vi "ex_SaveExcelFileCheckName.vi"(4 "file exists?":bool, 5 "overwrite_mode_multi":T2(ring)=enum."overwrite & backup", 6 "multi_file":bool, 7 "overwrite_mode":T3(ring), 8 "error in (no error)":errorcluster, 9 "enable file ops":bool, 11 "file path":path) -> (0 "error out":errorcluster, 2 "function":T1, 3 "file path out":path)   [LabVIEW 2017]
uses:
  <vilib>/express/express shared/NI_ExcelFile/Ctrls/FileOperation.ctl
  <vilib>/express/express shared/NI_ExcelFile/NI_ExcelFile.lvlib
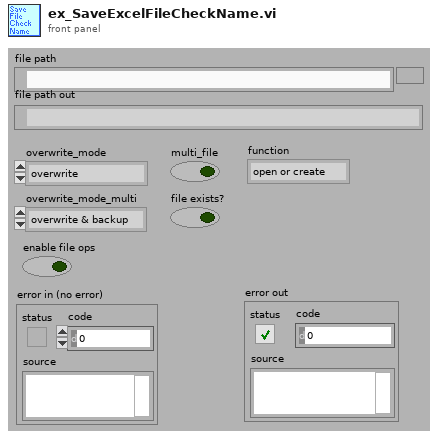
[diagram p1: front panel]
types:
  T1 = typedef "NI_ExcelFile.lvlib/FileOperation.ctl" = enum16{"open or create", "open", "create or replace", "create"}
  T2 = enum16{"overwrite", "overwrite & backup", "next avail"}
  T3 = enum16{"overwrite", "overwrite & backup", "append", "next avail"}
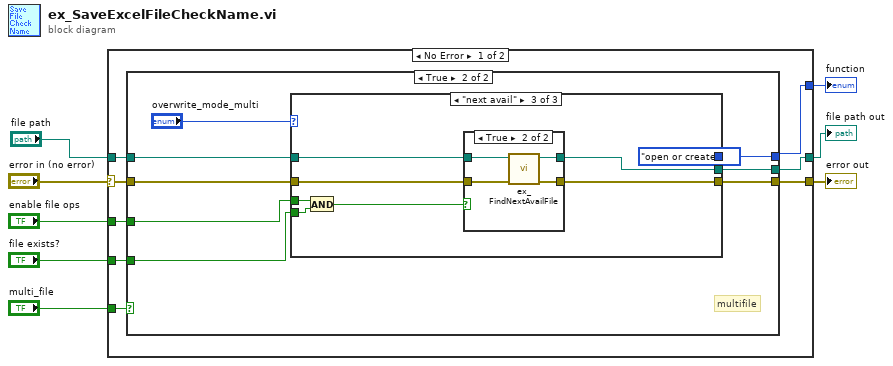
[diagram p0: block diagram]
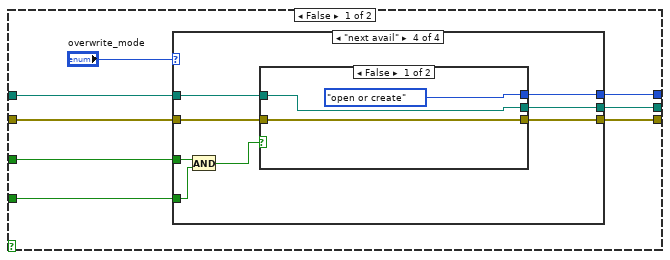
[diagram p2: hidden frame]
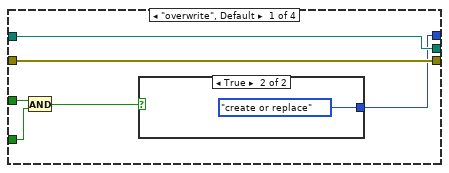
[diagram p3: hidden frame]
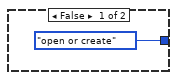
[diagram p4: hidden frame]
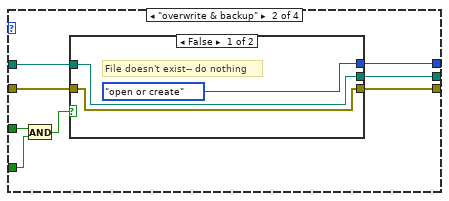
[diagram p5: hidden frame]
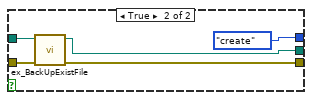
[diagram p6: hidden frame]
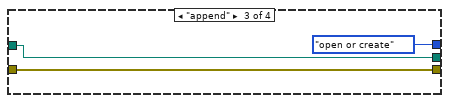
[diagram p7: hidden frame]
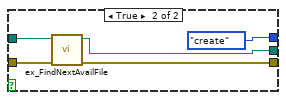
[diagram p8: hidden frame]
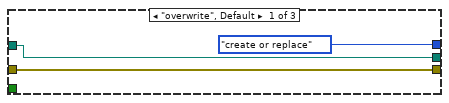
[diagram p9: hidden frame]
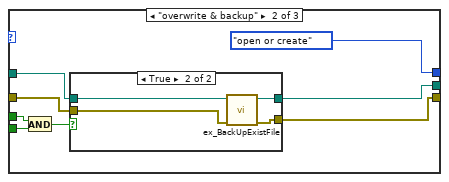
[diagram p10: hidden frame]
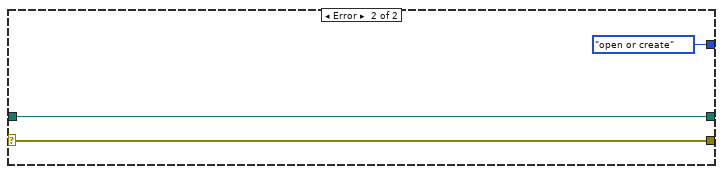
[diagram p13: hidden frame]
diagram:
  n1 = case shown="No Error" "error in (no error)" {
    selector: "error in (no error)" -> [w15 w109]
    tunnel: [w16 w109] -> w1
    tunnel: [w14 FileOperation."open or create" ("operation (0:open or create)")] -> w7
    tunnel: [w13 w107] -> w6
    tunnel: "multi_file" -> [w12 _]
    tunnel: "enable file ops" -> [w11 _]
    tunnel: "file exists?" -> [w10 _]
    tunnel: "file path" -> [w9 w107]
    frame No Error {
      n2 = case shown="True" w12 {
        tunnel: [w23 w74] -> w14
        tunnel: w9 -> [w18 w73]
        tunnel: [w20 w71] -> w13
        tunnel: [w19 w70] -> w16
        tunnel: w10 -> [w22 w69]
        tunnel: w15 -> [w21 w72]
        tunnel: w11 -> [w17 w68]
        frame False {
          n3 = case shown="\"next avail\"" "overwrite_mode" {
            tunnel: [w28 w33 FileOperation."open or create" ("operation (0:open or create)") w52] -> w23
            tunnel: w22 -> [w26 w34 _ w54]
            tunnel: w18 -> [w30 w38 w51 w59]
            tunnel: w21 -> [w29 w37 w49 w56]
            tunnel: [w30 w40 w51 w57] -> w20
            tunnel: [w29 w39 w49 w58] -> w19
            tunnel: w17 -> [w27 w35 _ w53]
            frame "overwrite", Default {
              n4 = And(x=w27, y=w26) -> (x .and. y?=w25:bool)
              n5 = case shown="True" w25 {
                tunnel: [FileOperation."open or create" ("operation (0:open or create)") FileOperation."create or replace" ("operation (0:open or create)")] -> w28
                frame False {
                }
                frame True {
                }
              }
            }
            frame "overwrite & backup" {
              n6 = And(x=w35, y=w34) -> (x .and. y?=w36:bool)
              n7 = case shown="False" w36 {
                tunnel: w38 -> [w42 w46]
                tunnel: w37 -> [w43 w45]
                tunnel: [w42 w48] -> w40
                tunnel: [w43 w47] -> w39
                tunnel: [FileOperation."open or create" ("operation (0:open or create)") FileOperation."create" ("operation (0:open or create)")] -> w33
                frame False {
                  # "File doesn't exist-- do nothing"
                }
                frame True {
                  n8 = call <vilib>:"ex_BackUpExistFile.vi"("error in"=w45, "file path"=w46) -> ("error out"=w47:errorcluster, "dup file path"=w48:path)  [unwired: 8 out]
                }
              }
            }
            frame "append" {
            }
            frame "next avail" {
              n9 = And(x=w53, y=w54) -> (x .and. y?=w55:bool)
              n10 = case shown="False" w55 {
                tunnel: w59 -> [w62 w67]
                tunnel: [w61 w66] -> w58
                tunnel: [w62 w65] -> w57
                tunnel: w56 -> [w61 w64]
                tunnel: [FileOperation."open or create" ("operation (0:open or create)") FileOperation."create" ("operation (0:open or create)")] -> w52
                frame False {
                }
                frame True {
                  n11 = call <vilib>:"ex_FindNextAvailFile.vi"("error in"=w64, "desired file path"=w67) -> ("error out"=w66:errorcluster, "next avail file path"=w65:path)  [unwired: 8 out]
                }
              }
            }
          }
        }
        frame True {
          # "multifile"
          n12 = case shown="\"next avail\"" "overwrite_mode_multi" {
            tunnel: [FileOperation."create or replace" ("operation (0:open or create)") FileOperation."open or create" ("operation (0:open or create)") FileOperation."open or create" ("operation (0:open or create)")] -> w74
            tunnel: w73 -> [w78 w86 w98]
            tunnel: w72 -> [w77 w85 w97]
            tunnel: [w78 w84 w100] -> w71
            tunnel: [w77 w83 w99] -> w70
            tunnel: w69 -> [_ w81 w95]
            tunnel: w68 -> [_ w80 w94]
            frame "overwrite", Default {
            }
            frame "overwrite & backup" {
              n13 = And(x=w80, y=w81) -> (x .and. y?=w82:bool)
              n14 = case shown="True" w82 {
                tunnel: w86 -> [w87 w90]
                tunnel: w85 -> [w88 w89]
                tunnel: [w87 w92] -> w84
                tunnel: [w88 w91] -> w83
                frame False {
                  # "File doesn't exist-- do nothing"
                }
                frame True {
                  n15 = call <vilib>:"ex_BackUpExistFile.vi"("error in"=w89, "file path"=w90) -> ("error out"=w91:errorcluster, "dup file path"=w92:path)  [unwired: 8 out]
                }
              }
            }
            frame "next avail" {
              n16 = And(x=w94, y=w95) -> (x .and. y?=w96:bool)
              n17 = case shown="True" w96 {
                tunnel: w98 -> [w102 w106]
                tunnel: [w101 w105] -> w99
                tunnel: [w102 w104] -> w100
                tunnel: w97 -> [w101 w103]
                frame False {
                }
                frame True {
                  n18 = call <vilib>:"ex_FindNextAvailFile.vi"("error in"=w103, "desired file path"=w106) -> ("error out"=w105:errorcluster, "next avail file path"=w104:path)  [unwired: 8 out]
                }
              }
            }
          }
        }
      }
    }
    frame Error {
    }
  }
  "function" <- w7
  "file path out" <- w6
  "error out" <- w1
